vi "Data Validation Example.vi"(8 "Passback Data":refnum<user-event>) -> ()   [LabVIEW 2020, in "Dialog Boxes.lvlib"]
uses:
  Dialog Boxes.lvlib
  toolbox/Data Manipulation/_polysubs/[true]=disable.vi
  toolbox/Data Manipulation/Data Manipulation.lvlib
  toolbox/User Interface/User Interface.lvlib
panel:
  out "output cluster":T1
  in  "Cancel":bool
  in  "Ok":bool
  in  "String 2":string
  in  "Numeric 2":dbl min=3.0 max=30.0
  in  "String 1":string
  in  "Numeric 1":dbl
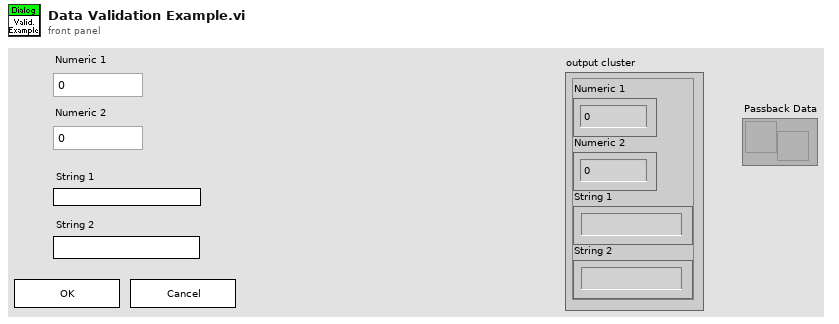
[diagram p1: front panel]
types:
  T1 = cluster{"Numeric 1":dbl, "Numeric 2":dbl, "String 1":string, "String 2":string}
  T2 = enum8{"Enabled", "Disabled", "Disabled and Grayed Out"}
  T3 = typedef "eventvkey.ctl" = enum16{"ASCII", "Enter", "Return", "Shift", "Ctrl", "Alt", "Cmd", "Opt", "Caps", "NumLock", "Clear", "Break", "Up", "Down", "Left", "Right", "Insert", "Delete", "Home", "End", "PageUp", "PageDown", "Escape", "Help", "Pause", "ScrollLock", "F1", "F2", "F3", "F4", "F5", "F6", "F7", "F8", "F9", "F10", "F11", "F12", "F13", "F14", "F15", "F16", "F17", "F18", "F19", "F20", "F21", "F22", "F23", "F24", "Play", "VolumeUp", "VolumeDown", "Mute", "Two Byte Char"}
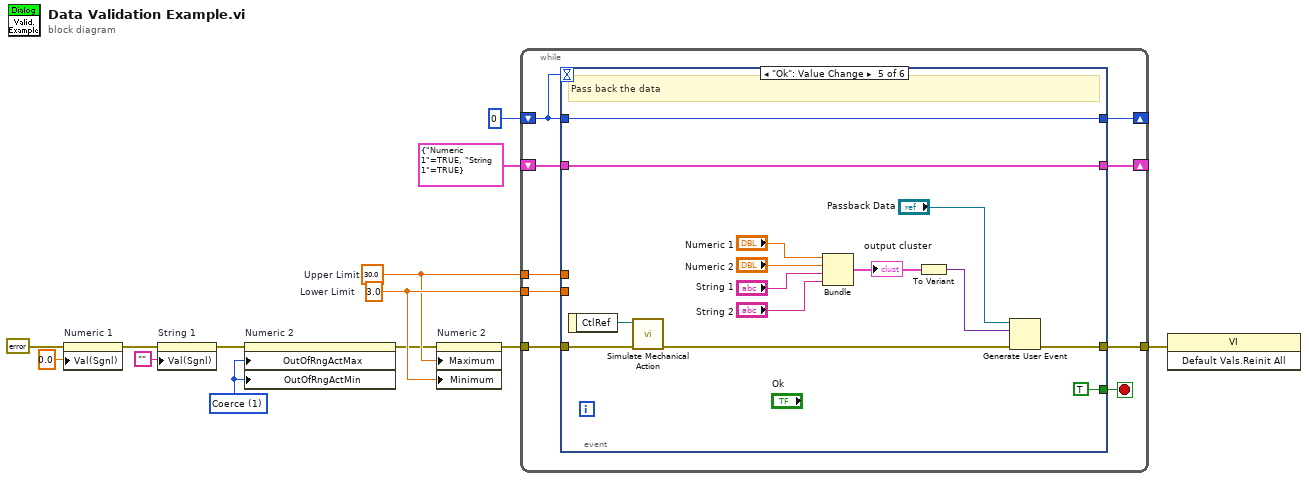
[diagram p0: block diagram]
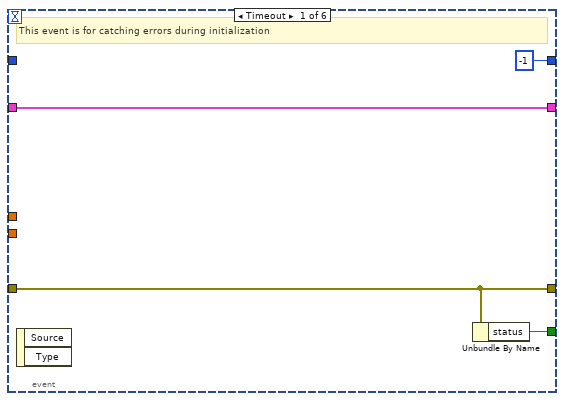
[diagram p2: hidden frame]
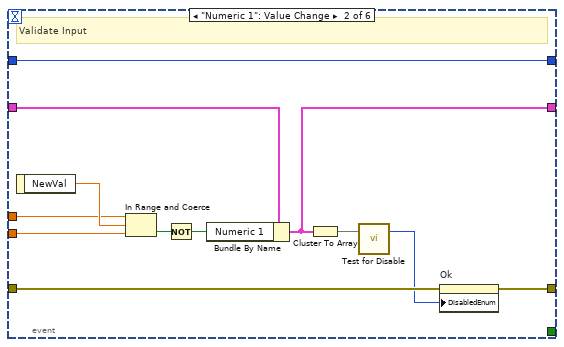
[diagram p3: hidden frame]
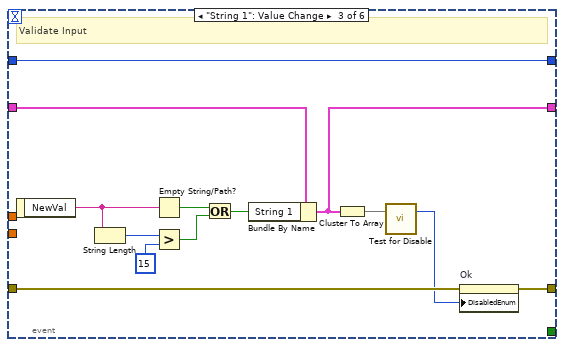
[diagram p4: hidden frame]
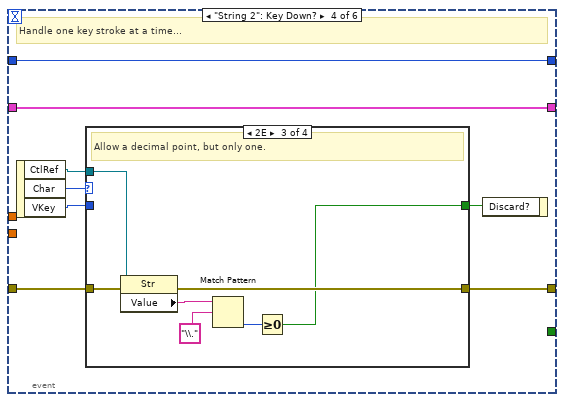
[diagram p5: hidden frame]
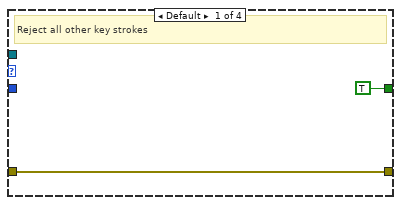
[diagram p6: hidden frame]
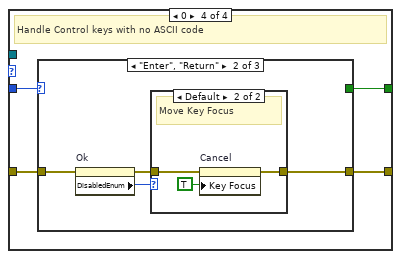
[diagram p8: hidden frame]
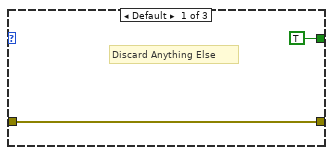
[diagram p9: hidden frame]
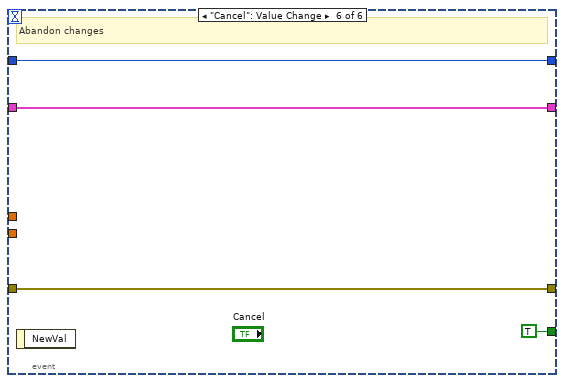
[diagram p12: hidden frame]
diagram:
  w7 = u8 1 items=["Ignore", "Coerce"] ("Response to Value Outside Limits:Minimum")
  w10 = 3.0  # Lower Limit
  w9 = 30.0  # Upper Limit
  n1 = property on="Numeric 1" class="DigNum (strict)"(error in=errorcluster {"status"=FALSE, "code"=0, "source"=""} ("error out"), "Val(Sgnl)"=0.0 ("Value (Signaling)")) -> (error out=w3:errorcluster)  [unwired: 1 in, 1 out]
  n2 = property on="String 1" class="Str"(error in=w3, "Val(Sgnl)"="") -> (error out=w2:errorcluster)  [unwired: 1 in, 1 out]
  n3 = property on="Numeric 2" class="DigNum (strict)"(error in=w2, "OutOfRngActMax"=w7, "OutOfRngActMin"=w7) -> (error out=w8:errorcluster)  [unwired: 1 in, 1 out]
  n4 = property on="Numeric 2" class="DigNum (strict)"(error in=w8, "Maximum"=w9, "Minimum"=w10) -> (error out=w11:errorcluster)  [unwired: 1 in, 1 out]
  n5 = while {
    shift-right: [w21] -> _
    shift-left: cluster{"Numeric 1":bool, "String 1":bool} {"Numeric 1"=TRUE, "String 1"=TRUE} -> [w20]
    tunnel: w11 -> [w19]
    tunnel: [w18] -> w1
    shift-right: [w17] -> _
    shift-left: 0 -> [w16]
    tunnel: w9 -> [w15]
    tunnel: w10 -> [w14]
    stop <- w22 stop-if-true
    n6 = event shown="[4] \"Ok\": Value Change" {
      selector: _ -> [_ _ _ _ _ _]
      dyn-events: _ -> [_ _ _ _ _ _]
      timeout: w16 -> [_ _ _ _ _ _]
      tunnel: [w23 _ _ _ TRUE TRUE] -> w22
      tunnel: [w26 w32 w45 w59 w96 w101] -> w21
      tunnel: w20 -> [w26 w33 w46 w59 w96 w101]
      tunnel: w19 -> [w24 w37 w50 w56 w90 w100]
      tunnel: [w24 w36 w49 w54 w87 w100] -> w18
      tunnel: w16 -> [_ w38 w51 w58 w97 w99]
      tunnel: [-1 w38 w51 w58 w97 w99] -> w17
      tunnel: w15 -> [_ w28 _ _ _ _]
      tunnel: w14 -> [_ w27 _ _ _ _]
      event Timeout {
        # "This event is for catching errors during initialization"
        n7 = event-data() -> ()  [unwired: 1 in, 2 out]
        n8 = Unbundle By Name(w24) -> ("status"=w23:bool)
      }
      event "Numeric 1": Value Change {
        # "Validate Input"
        n9 = event-data() -> ("NewVal"=w31:dbl)  [unwired: 1 in]
        n10 = In Range and Coerce(upper limit=w28, x=w31, lower limit=w27) -> (In Range?=w30:bool)  [unwired: 1 out]
        n11 = Not(x=w30) -> (.not. x?=w29:bool)
        n12 = Bundle By Name(cluster=w33, "Numeric 1"=w29) -> (w32:cluster{"Numeric 1":bool, "String 1":bool})
        n13 = Cluster To Array(cluster=w32) -> (array=w35:bool[])
        n14 = call-poly "Test for Disable.vi"("Flags"=w35) -> ("Disabled"=w34:T2)  [unwired: 2 in]
        n15 = property on="Ok" class="Bool (strict)"(error in=w37, "DisabledEnum"=w34) -> (error out=w36:errorcluster)  [unwired: 1 in, 1 out]
      }
      event "String 1": Value Change {
        # "Validate Input"
        n16 = event-data() -> ("NewVal"=w41:string)  [unwired: 1 in]
        n17 = String Length(string=w41) -> (length=w40:i32)
        n18 = Empty String/Path?(string/path=w41) -> (empty?=w43:bool)
        n19 = Greater?(x=w40, y=15) -> (0:w42:bool)
        n20 = Or(x=w43, y=w42) -> (x .or. y?=w44:bool)
        n21 = Bundle By Name(cluster=w46, "String 1"=w44) -> (w45:cluster{"Numeric 1":bool, "String 1":bool})
        n22 = Cluster To Array(cluster=w45) -> (array=w48:bool[])
        n23 = call-poly "Test for Disable.vi"("Flags"=w48) -> ("Disabled"=w47:T2)  [unwired: 2 in]
        n24 = property on="Ok" class="Bool (strict)"(error in=w50, "DisabledEnum"=w47) -> (error out=w49:errorcluster)  [unwired: 1 in, 1 out]
      }
      event "String 2": Key Down? {
        # "Handle one key stroke at a time..."
        n25 = event-data() -> ("CtlRef"=w53:refnum<vi>, "Char"=w57:i16, "VKey"=w52:T3)  [unwired: 1 in]
        n26 = case shown="2E" w57 {
          tunnel: w56 -> [w61 w62 w69 w72]
          tunnel: [TRUE _ w63 w73] -> w55
          tunnel: [w61 w62 w66 w71] -> w54
          tunnel: w53 -> [_ _ w68 _]
          tunnel: w52 -> [_ _ _ w70]
          frame Default {
            # "Reject all other key strokes"
          }
          frame 8, 9, 48..57 {
            # "Allow backspace, tab and digits 0 - 9"
          }
          frame 46 {
            # "Allow a decimal point, but only one."
            n27 = property class="Str"(reference=w68, error in=w69) -> (error out=w66:errorcluster, "Value"=w67:string)  [unwired: 1 out]
            n28 = Match Pattern(string=w67, regular expression="\\.") -> (offset past match=w64:i32)  [unwired: 1 in, 3 out]
            n29 = Greater Or Equal To 0?(x=w64) -> (x >= 0?=w63:bool)
          }
          frame 0 {
            # "Handle Control keys with no ASCII code"
            n30 = case shown="\"Enter\", \"Return\"" w70 {
              tunnel: [TRUE _ _] -> w73
              tunnel: w72 -> [w74 w79 w84]
              tunnel: [w74 w78 w84] -> w71
              frame Default {
                # "Discard Anything Else"
              }
              frame "Enter", "Return" {
                n31 = property on="Ok" class="Bool (strict)"(error in=w79) -> (error out=w77:errorcluster, "DisabledEnum"=w76:T2)  [unwired: 1 in, 1 out]
                n32 = case shown="Default" w76 {
                  tunnel: [w80 w81] -> w78
                  tunnel: w77 -> [w80 w82]
                  frame "Enabled" {
                    # "The button will click"
                  }
                  frame Default {
                    # "Move Key Focus"
                    n33 = property on="Cancel" class="Bool"(error in=w82, "Key Focus"=TRUE) -> (error out=w81:errorcluster)  [unwired: 1 in, 1 out]
                  }
                }
              }
              frame "Left", "Right", "Delete" {
              }
            }
          }
        }
        n34 = event-data("Discard?"=w55) -> ()  [unwired: 1 in, 1 out]
      }
      event "Ok": Value Change {
        # "Pass back the data"
        n35 = event-data() -> ("CtlRef"=w91:refnum<vi>)  [unwired: 1 in]
        n36 = call "Simulate Mechanical Action.vi"("Error In"=w90, "Button CtlRef"=w91) -> ("Error Out"=w88:errorcluster)  [unwired: 5 in]
        n37 = Bundle("Numeric 1"="Numeric 1", "Numeric 2"="Numeric 2", "String 1"="String 1", "String 2"="String 2") -> (w89:T1)  [unwired: 1 in]
        "output cluster" <- w89
        n38 = To Variant(anything=w89) -> (Variant=w86:variant)
        n39 = Generate User Event(user event="Passback Data", event data cluster=w86, error in=w88) -> (error out=w87:errorcluster)  [unwired: 1 in, 1 out]
      }
      event "Cancel": Value Change {
        # "Abandon changes"
        n40 = event-data() -> ()  [unwired: 1 in, 1 out]
      }
    }
  }
  n41 = invoke class="VI" method="Default Vals.Reinit All"(error in=w1) -> ()  [unwired: 2 in, 3 out]
